vi "Plot Editor Asynchronous Call.vi"(8 "error in (no error)":errorcluster, 10 "Coords":T1, 11 "XYGraph in":T2) -> (0 "Error Out":errorcluster, 1 "Message":string, 2 "Plot Name":string, 3 "Graph Caption":string)   [LabVIEW 2019, in "Plot Editor.lvlib"]
uses:
  Plot Editor.lvlib
  XY Graph Refnum.ctl
  <vilib>/Utility/miscctls.llb/LVPoint32TypeDef.ctl
  XY Graph Add-Ons.lvlib
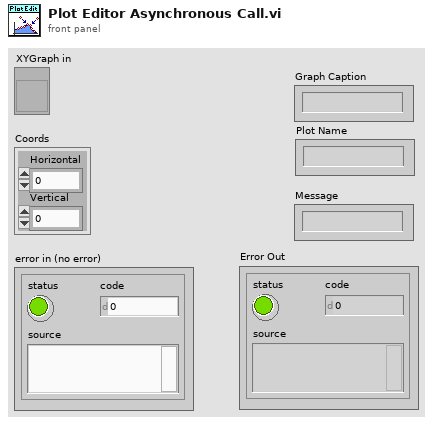
[diagram p1: front panel]
types:
  T1 = typedef "LVPoint32TypeDef.ctl" = cluster{"Horizontal":i32, "Vertical":i32}
  T2 = typedef "XY Graph Add-Ons.lvlib/XY Graph Refnum.ctl" = refnum<vi>
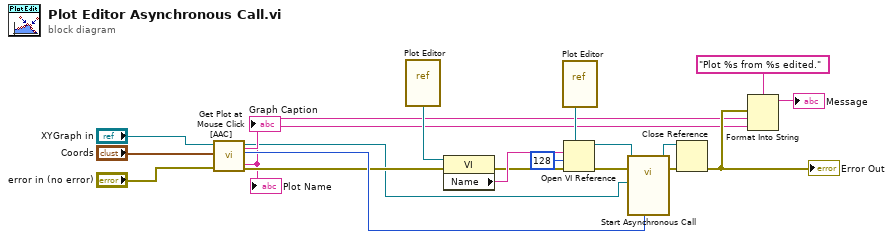
[diagram p0: block diagram]
diagram:
  n1 = call "Get Plot at Mouse Click [AAC].vi"("error in (no error)"="error in (no error)", "Mouse Click Coordinates"="Coords", "XYGraph Ref"="XYGraph in") -> ("error out"=w16:errorcluster, "Plot at Coordinates"=w20:i32, "XYGraph Ref"=w1:T2, "Plot Name"=w2:string, "Graph Caption"=w3:string)  [unwired: 2 in, 2 out]
  "Plot Name" <- w2
  "Graph Caption" <- w3
  n2 = vi-ref "Plot Editor.vi"() -> (w8:refnum<vi>)
  n3 = property class="VI"(reference=w8, error in=w16) -> (error out=w9:errorcluster, "Name"=w10:string)  [unwired: 1 out]
  n4 = vi-ref "Plot Editor.vi"() -> (w11:refnum<vi>)
  n5 = Open VI Reference(type specifier VI Refnum (for type only)=w11, vi path=w10, options=128, error in (no error)=w9) -> (vi reference=w14:refnum<vi>, error out=w15:errorcluster)  [unwired: 2 in]
  n6 = call-by-ref "Start Asynchronous Call"(reference=w14, error in=w15, "Original Plot Idx"=w20, "Original Graph Refnum"=w1) -> (reference out=w13:refnum<vi>, error out=w12:errorcluster)  [unwired: 7 in, 3 out]
  n7 = Close Reference(reference=w13, error in (no error)=w12) -> (error out=w6:errorcluster)
  "Error Out" <- w6
  n8 = Format Into String(format string="Plot %s from %s edited.", error in=w6, w2, w3) -> (resulting string=→"Message":string)  [unwired: 1 in, 1 out]
